vi "PicoScope3000aOpen.vi"(0 "error in (no error)":errorcluster, 1 "Serial Number":string, 2 "Mode":u16(ring) items=["Dialog On Error", "no dialog - CloseUnit and Stop", "no dialog - Continue", "no dialog - Stop"], 5 "Use Serial number":bool, 9 "USB 3.0 device on non-USB 3.0 Port Control":bool=TRUE, 11 "USB Powered Control":bool=TRUE) -> (3 "Pico 3000a Units":string, 4 "error out":errorcluster, 6 "handle":i16, 10 "USB Powered":bool=TRUE, 12 "Device Info":T1, 14 "Max ADC value":i16, 15 "USB 3.0 device on non-USB 3.0 Port":bool=TRUE)   [LabVIEW 2010]
doc: "This VI opens a PicoScope 3000a/b and returns a handle to the device."
uses:
  ps3000a.dll
panel:
  out "serialLth":i16
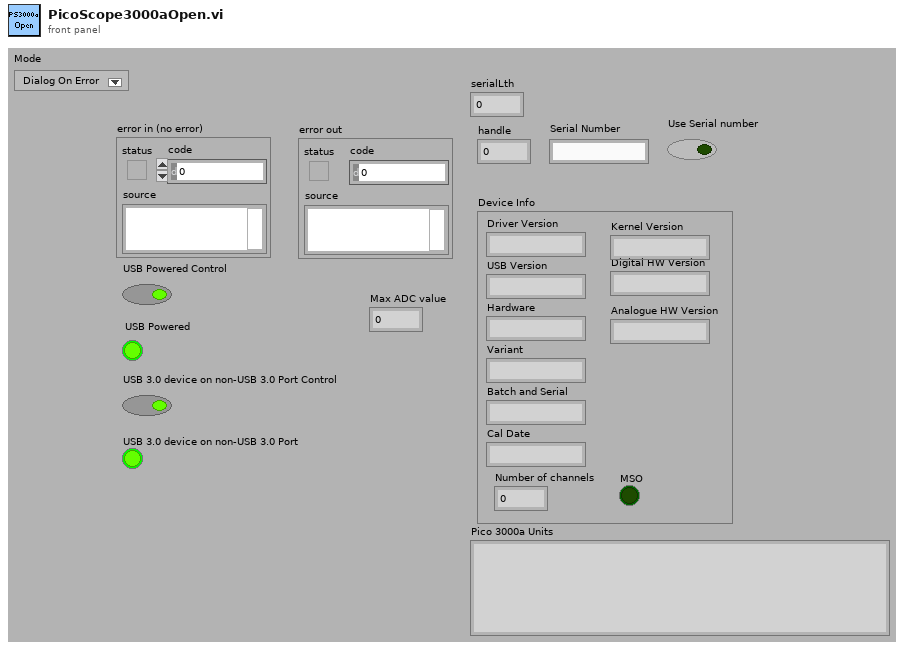
[diagram p1: front panel]
types:
  T1 = cluster{"Driver Version":string, "USB Version":string, "Hardware":string, "Variant":string, "Batch and Serial":string, "Cal Date":string, "Kernel Version":string, "Digital HW Version":string, "Analogue HW Version":string, "MSO":bool, "Number of channels":i16}
  T2 = cluster{"status":bool, "code":u32, "source":string}
  T3 = cluster{"Driver Version":string, "USB Version":string, "Hardware":string, "Variant":string, "Batch and Serial":string, "Cal Date":string, "Kernel Version":string, "Digital HW Version":string, "Analogue HW Version":string}
  T4 = cluster{"Driver Version":string, "USB Version":string, "Hardware":string, "Variant":string, "Batch and Serial":string, "Cal Date":string, "Kernel Version":string, "Digital HW Version":string, "Analogue HW Version":string, bool, i16}
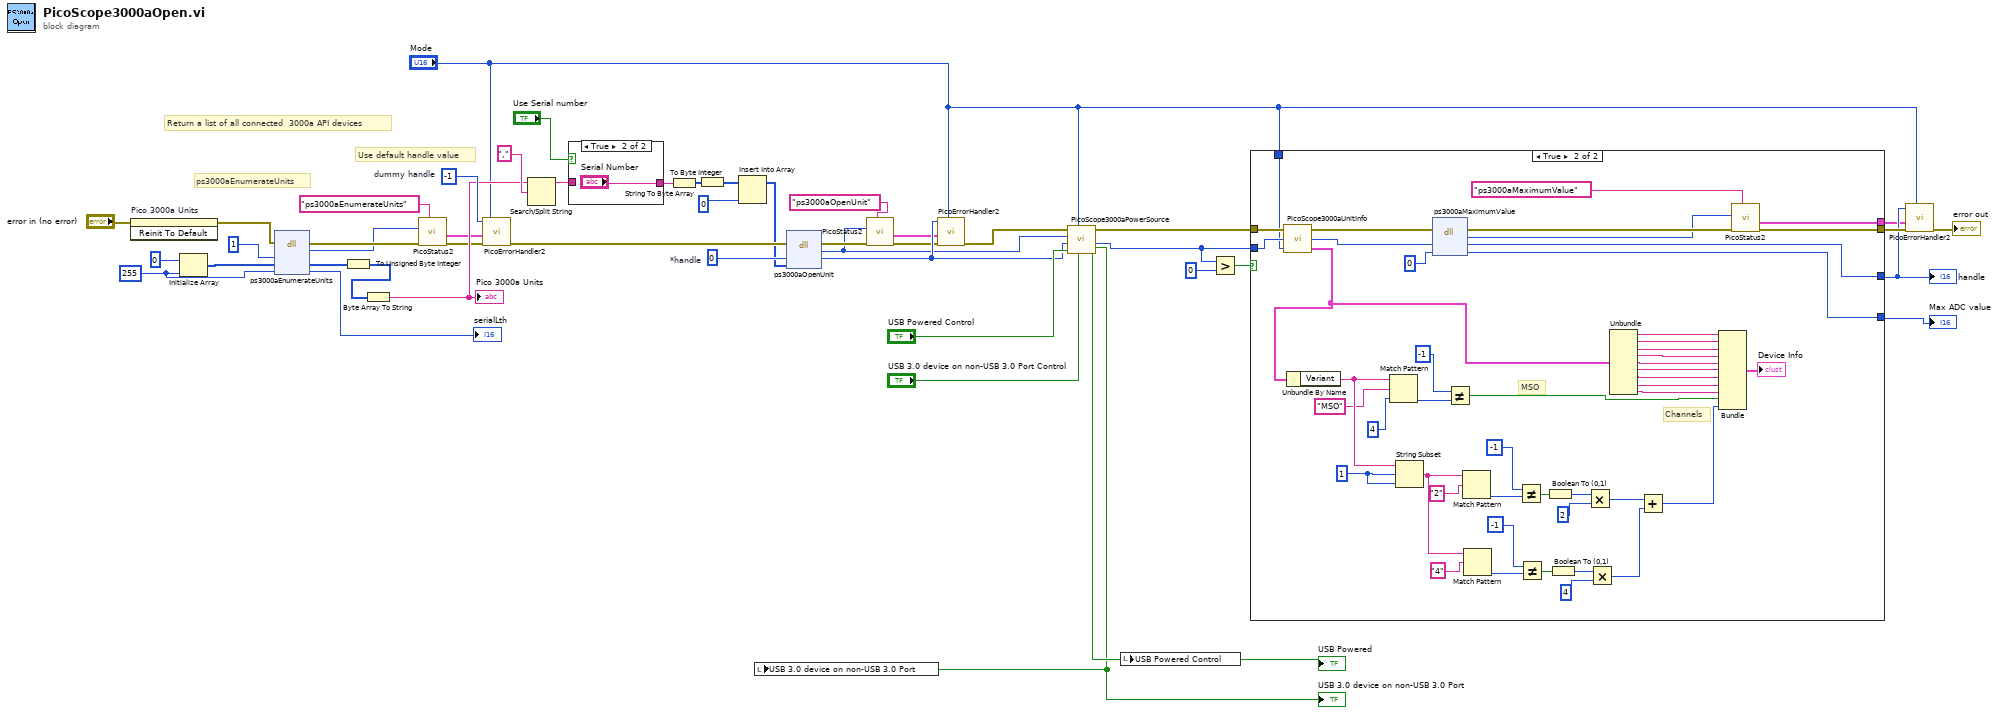
[diagram p0: block diagram]
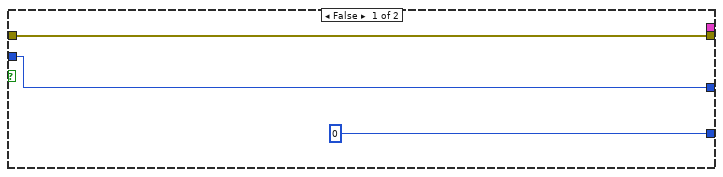
[diagram p3: hidden frame]
diagram:
  w24 = i16 -1  # dummy handle
  w28 = i16 255 ("dimension size")
  w33 = i16 0  # *handle
  # "Use default handle value"
  # "Return a list of all connected  3000a API devices"
  # "ps3000aEnumerateUnits"
  n1 = invoke on="Pico 3000a Units" class="Str" method="Reinit To Default"(error in="error in (no error)") -> (error out=w25:errorcluster)  [unwired: 2 in, 2 out]
  n2 = Initialize Array(i8 0 ("U8"), w28) -> (w30:i8[])
  n3 = dll-call lib="ps3000a.dll" fn="ps3000aEnumerateUnits"(error in=w25, "count"=i16 1, "serials"=w30, "serialLth"=w28) -> (error out=w10:errorcluster, "PICO_STATUS"=w9:u32, "serials"=w26:i8[], "serialLth"=→"serialLth":i16)  [unwired: 3 in, 1 out]
  n4 = To Unsigned Byte Integer(number=w26) -> (unsigned 8bit integer=w27:u8[])
  n5 = Byte Array To String(unsigned byte array=w27) -> (string=w14:string)
  "Pico 3000a Units" <- w14
  n6 = call "PicoStatus2.vi"("PICO source"="ps3000aEnumerateUnits" ("source"), "Error in"=w10, "PICO STATUS"=w9) -> ("error out"=w11:errorcluster, "PICO_STATUS out"=w8:T2)  [unwired: 5 in]
  n7 = call "PicoErrorHandler2.vi"("Mode"="Mode", "error in (no error)"=w11, "PICO_STATUS in"=w8, "handle In"=w24) -> ("error out"=w22:errorcluster)  [unwired: 7 in]
  n8 = Search/Split String(string=w14, search string/char (-)=",") -> (substring before match=w20:string)  [unwired: 1 in, 2 out]
  n9 = case shown="True" "Use Serial number" {
    tunnel: w20 -> [w48 _]
    tunnel: [w48 "Serial Number"] -> w16
    frame False {
    }
    frame True {
    }
  }
  n10 = String To Byte Array(string=w16) -> (unsigned byte array=w18:u8[])
  n11 = To Byte Integer(number=w18) -> (8bit integer=w19:i8[])
  n12 = Insert Into Array(array=w19, new element=i8 0 ("new element/subarray")) -> (w13:i8[])  [unwired: 1 in]
  n13 = dll-call lib="ps3000a.dll" fn="ps3000aOpenUnit" ("ps3000.dll:_ps3000_open_unit@0")(error in=w22, "handle"=w33, "serial"=w13) -> (error out=w7:errorcluster, "PICO_STATUS"=w4:u32, "handle"=w34:i16)  [unwired: 3 in, 1 out]
  n14 = call "PicoStatus2.vi"("PICO source"="ps3000aOpenUnit" ("source"), "Error in"=w7, "PICO STATUS"=w4) -> ("error out"=w6:errorcluster, "PICO_STATUS out"=w5:T2)  [unwired: 5 in]
  n15 = call "PicoErrorHandler2.vi"("Mode"="Mode", "error in (no error)"=w6, "PICO_STATUS in"=w5, "handle In"=w34) -> ("error out"=w38:errorcluster)  [unwired: 7 in]
  n16 = call "PicoScope3000aPowerSource.vi"("USB 3.0 on non-USB 3.0 port control"="USB 3.0 device on non-USB 3.0 Port Control", "Mode"="Mode", "USB Powered control"="USB Powered Control", "handle in"=w34, "PICO STATUS IN"=w4, "error in (no error)"=w38) -> ("USB Powered"=w46:bool, "handle out"=w42:i16, "error out"=w39:errorcluster, "USB 3.0 on non-USB 3.0 Port"=w44:bool)  [unwired: 1 in, 1 out]
  "USB Powered" <- w46
  "USB 3.0 device on non-USB 3.0 Port" <- w44
  n17 = local write "USB 3.0 device on non-USB 3.0 Port"(w44) -> ()
  n18 = local write "USB Powered Control"(w46) -> ()
  n19 = Greater?(x=w42, y=0) -> (0:w43:bool)
  n20 = case shown="True" w43 {
    tunnel: w42 -> [w51 w99]
    tunnel: w39 -> [w52 w98]
    tunnel: [w52 w57] -> w36
    tunnel: [w51 w96] -> w35
    tunnel: [i16 0 ("value") w95] -> w40
    tunnel: "Mode" -> [_ w58]
    tunnel: [_ w55] -> w1
    frame False {
    }
    frame True {
      w84 = 1 ("offset (0)")
      # "MSO"
      # "Channels"
      n21 = call "PicoScope3000aUnitInfo.vi"("Mode"=w58, "handle in"=w99, "error in (no error)"=w98) -> ("Unit Info"=w75:T3, "handle out"=w97:i16, "error out"=w59:errorcluster)
      n22 = Unbundle By Name(w75) -> ("Variant"=w80:string)
      n23 = Match Pattern(string=w80, regular expression="MSO", offset (0)=4) -> (offset past match=w77:i32)  [unwired: 3 out]
      n24 = String Subset(string=w80, offset (0)=w84, length (rest)=w84) -> (substring=w70:string)
      n25 = dll-call lib="ps3000a.dll" fn="ps3000aMaximumValue"(error in=w59, "handle"=w97, "value"=i16 0) -> (error out=w56:errorcluster, "PICO_STATUS"=w53:u32, "handle"=w96:i16, "value"=w95:i16)  [unwired: 2 in, 1 out]
      n26 = Not Equal?(x=-1, y=w77) -> (x != y?=w74:bool)
      n27 = Match Pattern(string=w70, regular expression="2") -> (offset past match=w82:i32)  [unwired: 1 in, 3 out]
      n28 = Match Pattern(string=w70, regular expression="4") -> (offset past match=w72:i32)  [unwired: 1 in, 3 out]
      n29 = Not Equal?(x=-1, y=w82) -> (x != y?=w66:bool)
      n30 = Not Equal?(x=-1, y=w72) -> (x != y?=w62:bool)
      n31 = Boolean To (0,1)(Boolean=w66) -> (0, 1=w65:i16)
      n32 = Boolean To (0,1)(Boolean=w62) -> (0, 1=w63:i16)
      n33 = Multiply(x=w65, y=i16 2) -> (x*y=w69:i16)
      n34 = Multiply(x=w63, y=i16 4) -> (x*y=w61:i16)
      n35 = Unbundle(w75) -> ("Driver Version"=w93:string, "USB Version"=w92:string, "Hardware"=w91:string, "Variant"=w90:string, "Batch and Serial"=w89:string, "Cal Date"=w88:string, "Kernel Version"=w87:string, "Digital HW Version"=w86:string, "Analogue HW Version"=w85:string)
      n36 = Add(x=w69, y=w61) -> (x+y=w68:i16)
      n37 = Bundle("Driver Version"=w93, "USB Version"=w92, "Hardware"=w91, "Variant"=w90, "Batch and Serial"=w89, "Cal Date"=w88, "Kernel Version"=w87, "Digital HW Version"=w86, "Analogue HW Version"=w85, w74, w68) -> (→"Device Info":T4)  [unwired: 1 in]
      n38 = call "PicoStatus2.vi"("PICO source"="ps3000aMaximumValue" ("source"), "Error in"=w56, "PICO STATUS"=w53) -> ("error out"=w57:errorcluster, "PICO_STATUS out"=w55:T2)  [unwired: 5 in]
    }
  }
  "handle" <- w35
  "Max ADC value" <- w40
  n39 = call "PicoErrorHandler2.vi"("Mode"="Mode", "error in (no error)"=w36, "PICO_STATUS in"=w1, "handle In"=w35) -> ("error out"=→"error out":errorcluster)  [unwired: 7 in]
